vi "lvssh2_session_callback_events_init.vi"(8 "error in (no error)":errorcluster, 11 "abstract":T1) -> (0 "error out":errorcluster, 3 "events":T2)   [LabVIEW 2017, in "libssh2.lvlib"]
doc: "Initialize abstract for lvssh2."
uses:
  libssh2.lvlib
  lvssh2_session_callback_events.ctl
  lvssh2_session_callback_send_function_input_args_32.ctl
  lvssh2_session_callback_receive_function_input_args_32.ctl
  lvssh2_userauth_keyboard_interactive_response_function_input_args_32.ctl
  lvssh2_session_callback_send_function_input_args_64.ctl
  lvssh2_session_callback_receive_function_input_args_64.ctl
  lvssh2_userauth_keyboard_interactive_response_function_input_args_64.ctl
  libssh2_session_abstract.ctl
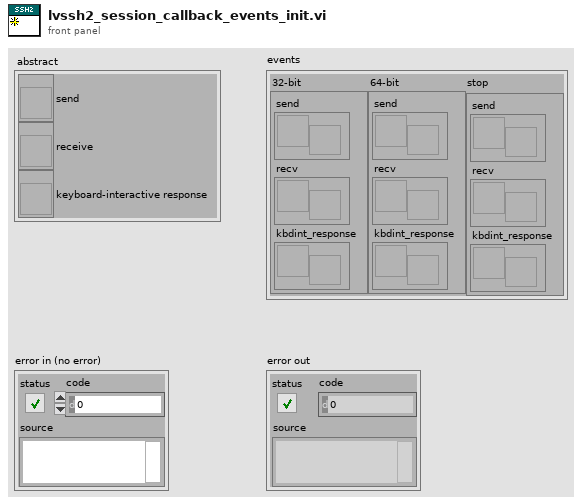
[diagram p1: front panel]
types:
  T1 = typedef "libssh2.lvlib/libssh2_session_abstract.ctl" = cluster{"send":refnum<vi>, "receive":refnum<vi>, "keyboard-interactive response":refnum<vi>}
  T2 = typedef "libssh2.lvlib/lvssh2_session_callback_events.ctl" = cluster{"32-bit":cluster{"send":refnum<user-event>, "recv":refnum<user-event>, "kbdint_response":refnum<user-event>}, "64-bit":cluster{"send":refnum<user-event>, "recv":refnum<user-event>, "kbdint_response":refnum<user-event>}, "stop":cluster{"send":refnum<user-event>, "recv":refnum<user-event>, "kbdint_response":refnum<user-event>}}
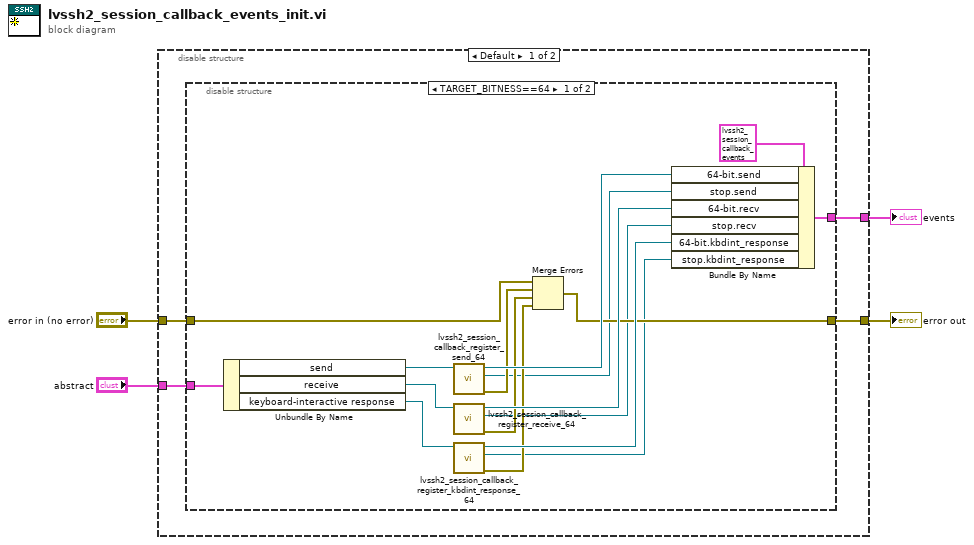
[diagram p0: block diagram]
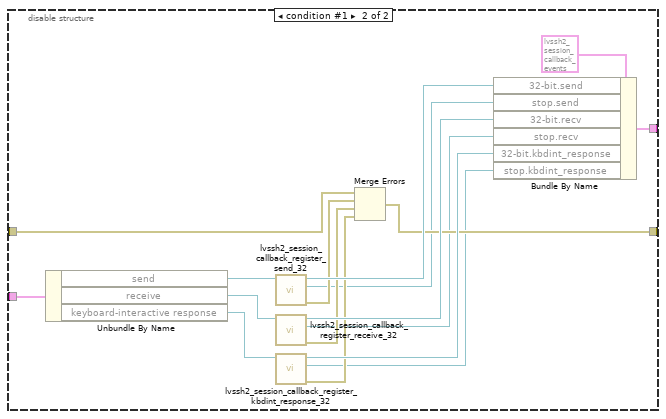
[diagram p2: hidden frame]
diagram:
  n1 = disable-structure shown="Default" {
    disable-tunnel: [w8 w43] -> w4
    disable-tunnel: "error in (no error)" -> [w7 w43]
    disable-tunnel: [w6 _] -> w2
    disable-tunnel: "abstract" -> [w5 _]
    frame condition #0 (active) {
      n2 = disable-structure shown="TARGET_BITNESS==64" {
        disable-tunnel: [w12 w29] -> w8
        disable-tunnel: w7 -> [w22 w39]
        disable-tunnel: [w25 w42] -> w6
        disable-tunnel: w5 -> [w23 w40]
        frame condition #0 (active) {
          n3 = Unbundle By Name(w23) -> ("send"=w21:refnum<vi>, "receive"=w18:refnum<vi>, "keyboard-interactive response"=w15:refnum<vi>)
          n4 = call "lvssh2_session_callback_register_send_64.vi"("send"=w21) -> ("error out"=w19:errorcluster, "stop event"=w10:refnum<user-event>, "user event"=w20:refnum<user-event>)  [unwired: 8 in]
          n5 = call "lvssh2_session_callback_register_receive_64.vi"("receive"=w18) -> ("error out"=w16:errorcluster, "stop event"=w9:refnum<user-event>, "user event"=w17:refnum<user-event>)  [unwired: 8 in]
          n6 = call "lvssh2_session_callback_register_kbdint_response_64.vi"("keyboard-interactive response"=w15) -> ("error out"=w13:errorcluster, "stop event"=w11:refnum<user-event>, "user event"=w14:refnum<user-event>)  [unwired: 8 in]
          n7 = Merge Errors(w22, w19, w16, w13) -> (w12:errorcluster)
          n8 = Bundle By Name(cluster=T2 {"32-bit"={"send"=refnum, "recv"=refnum, "kbdint_response"=refnum}, "64-bit"={"send"=refnum, "recv"=refnum, "kbdint_response"=refnum}, "stop"={"send"=refnum, "recv"=refnum, "kbdint_response"=refnum}} ("events"), "64-bit.send"=w20, "stop.send"=w10, "64-bit.recv"=w17, "stop.recv"=w9, "64-bit.kbdint_response"=w14, "stop.kbdint_response"=w11) -> (w25:T2)
        }
        frame condition #1 {
          n9 = Unbundle By Name(w40) -> ("send"=w38:refnum<vi>, "receive"=w35:refnum<vi>, "keyboard-interactive response"=w32:refnum<vi>)
          n10 = call "lvssh2_session_callback_register_send_32.vi"("send"=w38) -> ("error out"=w36:errorcluster, "stop event"=w27:refnum<user-event>, "user event"=w37:refnum<user-event>)  [unwired: 8 in]
          n11 = call "lvssh2_session_callback_register_receive_32.vi"("receive"=w35) -> ("error out"=w33:errorcluster, "stop event"=w26:refnum<user-event>, "user event"=w34:refnum<user-event>)  [unwired: 8 in]
          n12 = call "lvssh2_session_callback_register_kbdint_response_32.vi"("keyboard-interactive response"=w32) -> ("error out"=w30:errorcluster, "stop event"=w28:refnum<user-event>, "user event"=w31:refnum<user-event>)  [unwired: 8 in]
          n13 = Merge Errors(w39, w36, w33, w30) -> (w29:errorcluster)
          n14 = Bundle By Name(cluster=T2 {"32-bit"={"send"=refnum, "recv"=refnum, "kbdint_response"=refnum}, "64-bit"={"send"=refnum, "recv"=refnum, "kbdint_response"=refnum}, "stop"={"send"=refnum, "recv"=refnum, "kbdint_response"=refnum}} ("events"), "32-bit.send"=w37, "stop.send"=w27, "32-bit.recv"=w34, "stop.recv"=w26, "32-bit.kbdint_response"=w31, "stop.kbdint_response"=w28) -> (w42:T2)
        }
      }
    }
    frame condition #1 {
    }
  }
  "error out" <- w4
  "events" <- w2
